vi "Roulette.vi"(11 "Range":cluster{dbl, dbl}[](array[cluster])) -> (3 "Index":i32)   [LabVIEW 2015, in "TSP Library.lvlib"]
uses:
  TSP Library.lvlib
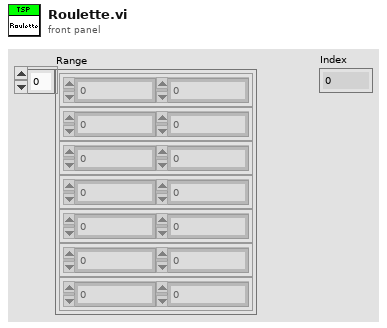
[diagram p1: front panel]
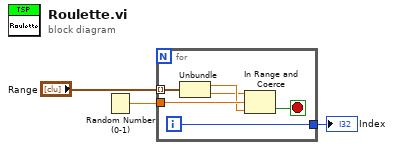
[diagram p0: block diagram]
diagram:
  n1 = Random Number (0-1)() -> (number: 0 to 1=w3:dbl)
  n2 = for {
    tunnel: "Range" -> [w6] mode=indexing
    tunnel: [w9] -> w1
    tunnel: w3 -> [w8]
    i -> [w9]
    stop <- w7 stop-if-true
    n3 = Unbundle(w6) -> (w5:dbl, w4:dbl)
    n4 = In Range and Coerce(upper limit=w4, x=w8, lower limit=w5) -> (In Range?=w7:bool)  [unwired: 1 out]
  }
  "Index" <- w1
